vi "IEEE574转浮点.vi"(1 "2_byte":i32 format="%0x", 2 "1_byte":i32 format="%x") -> (0 "Outvalue":dbl)   [LabVIEW 2016]
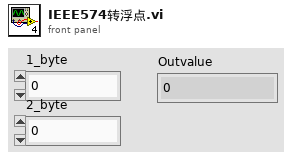
[diagram p1: front panel]
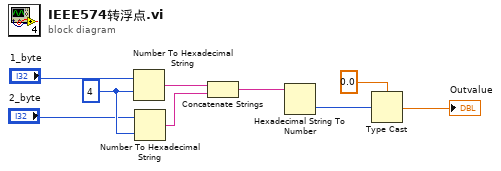
[diagram p0: block diagram]
diagram:
  w3 = i16 4 ("宽度(-)")
  n1 = Number To Hexadecimal String(1:w3, 2:"1_byte") -> (0:w5:string)
  n2 = Number To Hexadecimal String(1:w3, 2:"2_byte") -> (0:w4:string)
  n3 = Concatenate Strings(w5, w4) -> (w6:string)
  n4 = Hexadecimal String To Number(string=w6) -> (number=w8:u32)  [unwired: 2 in, 1 out]
  n5 = Type Cast(type=sgl 0.0, x=w8) -> (*(type *) &x=→"Outvalue":sgl)
